vi "GET-MKR.vi"(6 "Timeout":u32=3000, 8 "error in":errorcluster {"code" format="%.0x"}, 11 "Session In":refnum<visa-resource-name>="GPIB0::16::INSTR") -> (0 "error out":errorcluster {"code" format="%.0x"}, 1 "Val1,Val2":dbl[](array[numeric]), 3 "Session Out":refnum<visa-resource-name>)   [LabVIEW 2018]
doc: "OUTPMARK will activate a marker if a marker is not already selected. It will also insure\nthat any current marker searches have been completed before transmitting data."
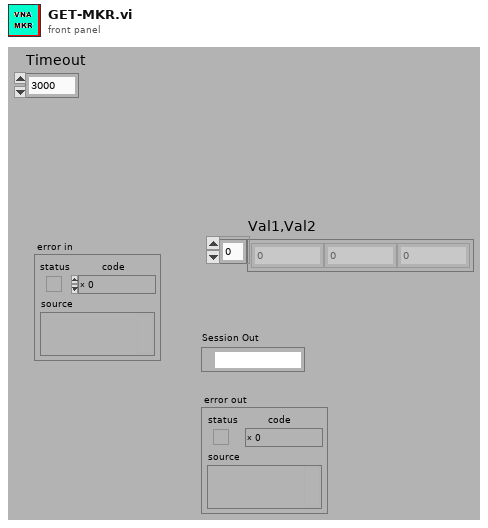
[diagram p1: front panel]
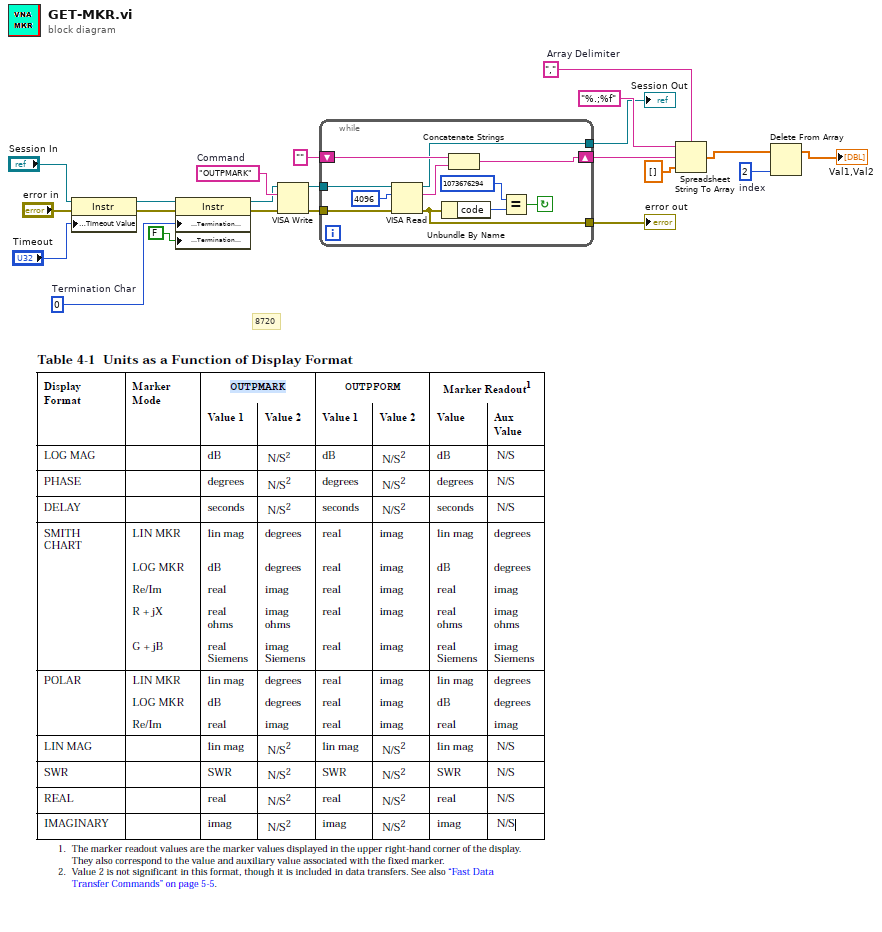
[diagram p0: block diagram]
diagram:
  w2 = 2  # index
  w7 = ","  # Array Delimiter
  w10 = "OUTPMARK"  # Command
  w17 = u8 0  # Termination Char
  # "8720"
  n1 = property class="Instr"(reference="Session In", error in="error in", "General Settings:Timeout Value"="Timeout") -> (reference out=w16:refnum<visa-resource-name>, error out=w19:errorcluster)
  n2 = property class="Instr"(reference=w16, error in=w19, "Message Based Settings:Termination Character"=w17, "Message Based Settings:Termination Character Enable"=FALSE ("enable")) -> (reference out=w5:refnum<visa-resource-name>, error out=w18:errorcluster)
  n3 = VISA Write(VISA resource name=w5, write buffer=w10, error in (no error)=w18) -> (VISA resource name out=w14:refnum<visa-resource-name>, error out=w13:errorcluster)  [unwired: 1 out]
  n4 = while {
    tunnel: w14 -> [w30]
    shift-right: [w24] -> w6
    shift-left: "" -> [w29]
    tunnel: w13 -> [w27]
    tunnel: [w26] -> w12
    tunnel: [w23] -> w4
    stop <- w25 continue-if-true
    n5 = VISA Read(VISA resource name=w30, byte count=u32 4096 ("byte count (0)"), error in (no error)=w27) -> (VISA resource name out=w23:refnum<visa-resource-name>, read buffer=w28:string, error out=w26:errorcluster)  [unwired: 1 out]
    n6 = Unbundle By Name(w26) -> ("code"=w32:i32)
    n7 = Concatenate Strings(w29, w28) -> (w24:string)
    n8 = Equal?(x=1073676294, y=w32) -> (x = y?=w25:bool)
  }
  "error out" <- w12
  "Session Out" <- w4
  n9 = Spreadsheet String To Array(delimiter (Tab)=w7, format string="%.;%f", spreadsheet string=w6, array type (2D Dbl)=dbl[] []) -> (array=w3:dbl[])
  n10 = Delete From Array(array=w3, index=w2) -> (array with subset deleted=→"Val1,Val2":dbl[])  [unwired: 1 in, 1 out]
